vi "Read Inputs from system.vi"(8 "error in":errorcluster, 11 "ActiveFrontEndModule runtime in":refnum<class "ActiveFrontEndModule runtime.lvclass">) -> (0 "error out":errorcluster, 2 "Inputs from system":T1, 3 "ActiveFrontEndModule runtime out":refnum<class "ActiveFrontEndModule runtime.lvclass">)   [LabVIEW 2017, in "ActiveFrontEndModule runtime.lvclass"]
uses:
  ActiveFrontEndModule runtime.lvclass
  configuration/input data indices.ctl
  ActiveFrontEndModule runtime.lvclass/ActiveFrontEndModule runtime.ctl
  configuration/ActiveFrontEndModule configuration.lvclass
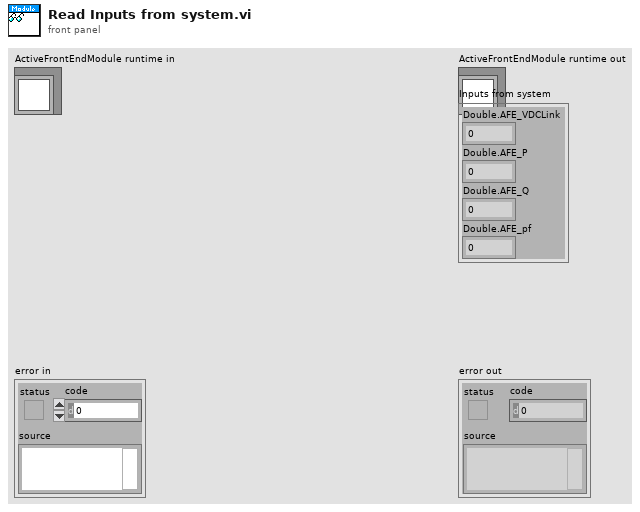
[diagram p1: front panel]
types:
  T1 = typedef "ActiveFrontEndModule configuration.lvclass/input data indices.ctl" = cluster{"Double.AFE_VDCLink":i32, "Double.AFE_P":i32, "Double.AFE_Q":i32, "Double.AFE_pf":i32}
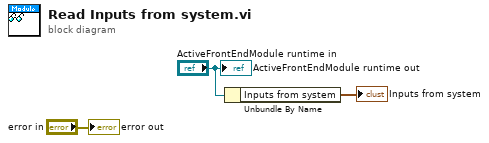
[diagram p0: block diagram]
diagram:
  n1 = Unbundle By Name("ActiveFrontEndModule runtime in") -> ("Inputs from system"=→"Inputs from system":T1)
  "error out" <- "error in"
  "ActiveFrontEndModule runtime out" <- "ActiveFrontEndModule runtime in"
